vi "SetLanguage.vi"(8 "error in (no error)":errorcluster, 10 "Language":string, 11 "FencedCodeBlock in":refnum<class "FencedCodeBlock.lvclass">) -> (0 "error out":errorcluster, 3 "FencedCodeBlock out":refnum<class "FencedCodeBlock.lvclass">)   [LabVIEW 2021, in "LvMarkdown.lvlib" / "FencedCodeBlock.lvclass"]
uses:
  FencedCodeBlock.lvclass
  FencedCodeBlock.lvclass/FencedCodeBlock.ctl
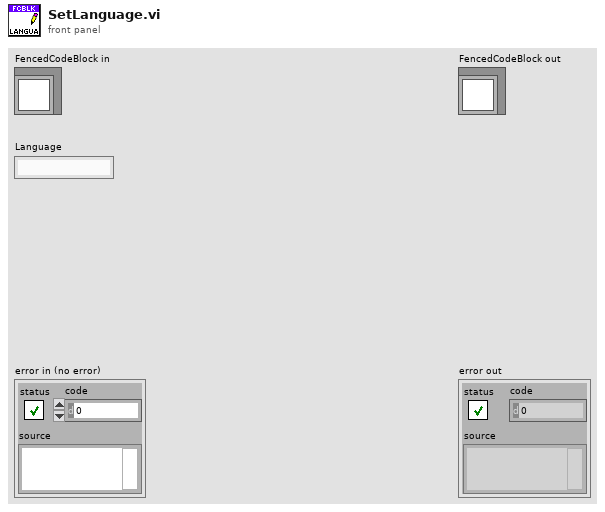
[diagram p1: front panel]
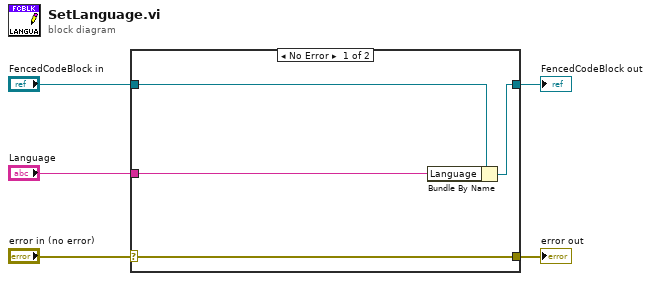
[diagram p0: block diagram]
diagram:
  n1 = case shown="No Error" "error in (no error)" {
    selector: "error in (no error)" -> [w9 w10]
    tunnel: [w9 w10] -> w4
    tunnel: [w7 w11] -> w2
    tunnel: "FencedCodeBlock in" -> [w8 w11]
    tunnel: "Language" -> [w6 _]
    frame No Error {
      n2 = Bundle By Name(cluster=w8, "Language"=w6) -> (w7:refnum<class "FencedCodeBlock.lvclass">)
    }
    frame Error {
    }
  }
  "error out" <- w4
  "FencedCodeBlock out" <- w2
